vi "Write target.vi"(8 "error in (no error)":errorcluster, 10 "GWTargetPositionParameters.lvclass":refnum<class "GWTargetPositionParameters.lvclass">, 11 "GuideTargetPosition in":refnum<class "GuideTargetPosition.lvclass">) -> (0 "error out":errorcluster, 3 "GuideTargetPosition out":refnum<class "GuideTargetPosition.lvclass">)   [LabVIEW 2014, in "TCSDataDefinitions.lvlib" / "TCSGuiderStatus.lvlib" / "GuideTargetPosition.lvclass"]
uses:
  GuideTargetPosition.lvclass
  GWTargetPositionParameters/GWTargetPositionParameters.lvclass
  GuideTargetPosition.lvclass/GuideTargetPosition.ctl
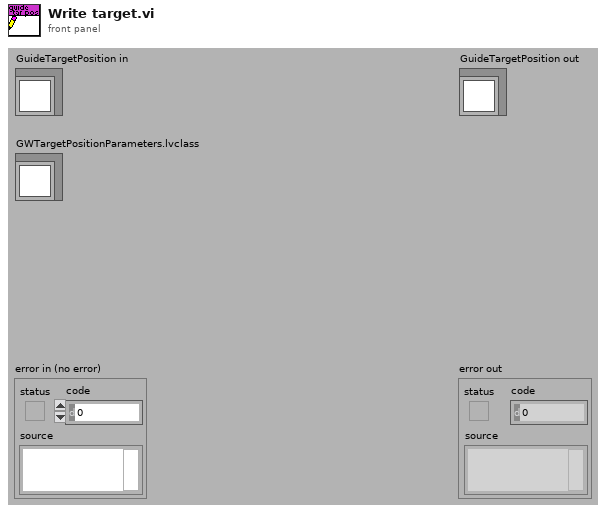
[diagram p1: front panel]
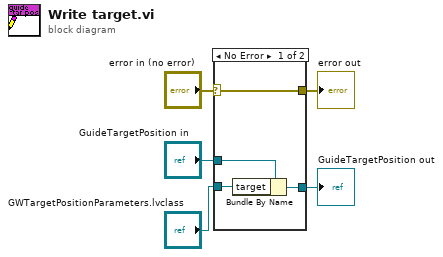
[diagram p0: block diagram]
diagram:
  n1 = case shown="No Error" "error in (no error)" {
    selector: "error in (no error)" -> [w9 w10]
    tunnel: [w9 w10] -> w4
    tunnel: [w7 w11] -> w2
    tunnel: "GuideTargetPosition in" -> [w8 w11]
    tunnel: "GWTargetPositionParameters.lvclass" -> [w6 _]
    frame No Error {
      n2 = Bundle By Name(cluster=w8, "target"=w6) -> (w7:refnum<class "GuideTargetPosition.lvclass">)
    }
    frame Error {
    }
  }
  "error out" <- w4
  "GuideTargetPosition out" <- w2
